vi "SubVi.vi"(11 "SubVi":refnum<queue>) -> ()   [LabVIEW 2012]
uses:
  States SubVi.ctl
panel:
  out "Waveform Chart":dbl(graph)
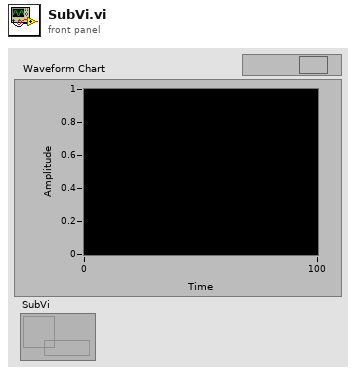
[diagram p1: front panel]
types:
  T1 = typedef "States SubVi.ctl" = enum16{"def", "Random", "Exit"}
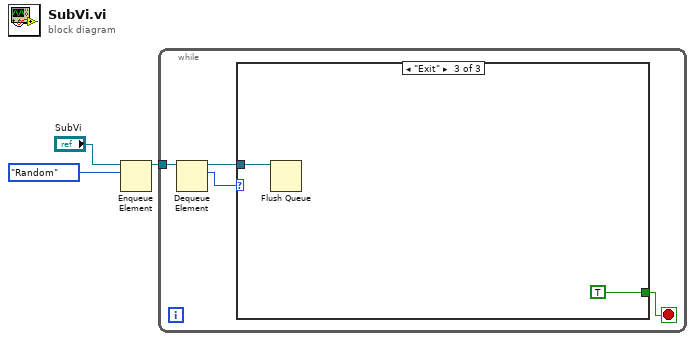
[diagram p0: block diagram]
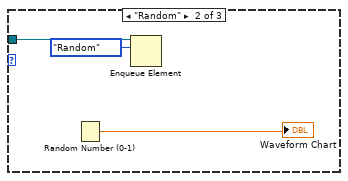
[diagram p3: hidden frame]
diagram:
  n1 = Enqueue Element(queue="SubVi", element=States_SubVi."Random") -> (queue out=w3:refnum<queue>)  [unwired: 2 in, 2 out]
  n2 = while {
    tunnel: w3 -> [w7]
    stop <- w4 stop-if-true
    n3 = Dequeue Element(queue=w7) -> (queue out=w5:refnum<queue>, element=w6:T1)  [unwired: 2 in, 2 out]
    n4 = case shown="\"Exit\"" w6 {
      tunnel: w5 -> [_ w9 w12]
      tunnel: [_ _ TRUE] -> w4
      frame "def", Default {
      }
      frame "Random" {
        n5 = Random Number (0-1)() -> (number: 0 to 1=→"Waveform Chart":dbl)
        n6 = Enqueue Element(queue=w9, element=States_SubVi."Random") -> ()  [unwired: 2 in, 3 out]
      }
      frame "Exit" {
        n7 = Flush Queue(queue=w12) -> ()  [unwired: 1 in, 3 out]
      }
    }
  }
